vi "Save Data-Complete.vi"(0 "SGP Array":dbl[](array[numeric]), 1 "Which Button?":T1(ring)=enum."Center Button", 5 "PTP Array":dbl[](array[numeric]), 9 "selected path":path, 11 "error in (no error)":errorcluster) -> (15 "error out":errorcluster)   [LabVIEW 2013]
panel:
  out "Header":string
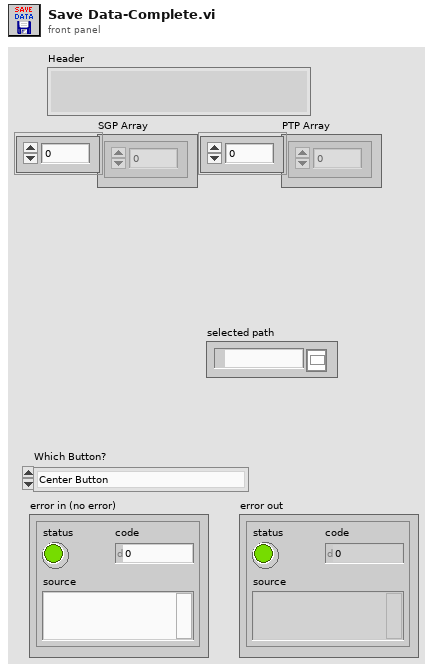
[diagram p1: front panel]
types:
  T1 = enum16{"Left Button", "Center Button", "Right Button", "Window Close"}
  T2 = enum16{"open", "replace", "create", "open or create", "replace or create", "replace or create with confirmation"}
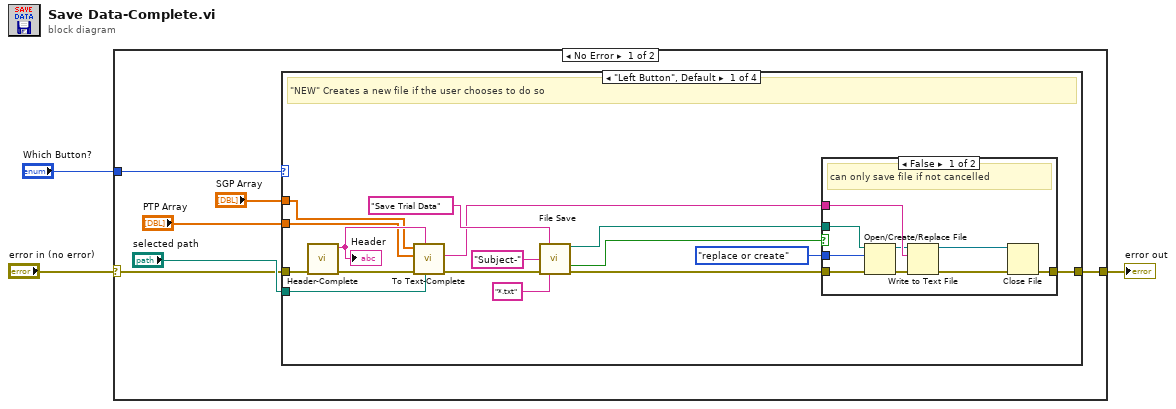
[diagram p0: block diagram]
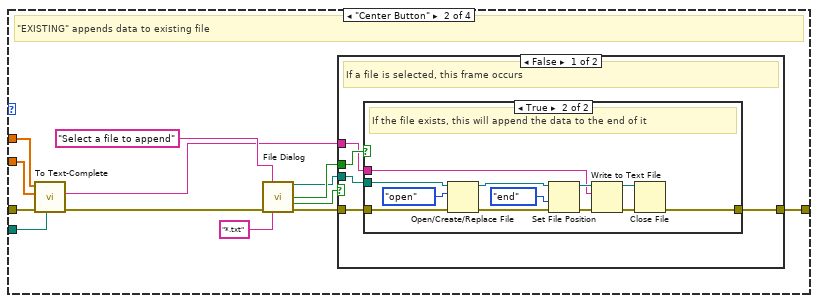
[diagram p3: hidden frame]
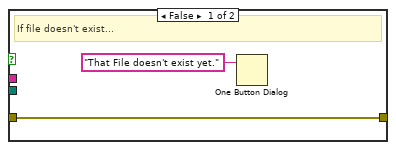
[diagram p4: hidden frame]
diagram:
  n1 = case shown="No Error" "error in (no error)" {
    selector: "error in (no error)" -> [w7 w71]
    tunnel: [w9 w71] -> w3
    tunnel: "Which Button?" -> [w6 _]
    frame No Error {
      n2 = case shown="\"Left Button\", Default" w6 {
        tunnel: w7 -> [w18 w39 w69 w70]
        tunnel: [w21 w45 w69 w70] -> w9
        tunnel: "selected path" -> [w15 w38 _ _]
        tunnel: "SGP Array" -> [w11 w37 _ _]
        tunnel: "PTP Array" -> [w10 w36 _ _]
        frame "Left Button", Default {
          # "\"NEW\" Creates a new file if the user chooses to do so"
          n3 = call "Header-Complete.vi"("error in (no error)"=w18) -> ("error out"=w16:errorcluster, "Headers"=w12:string)  [unwired: 9 in]
          "Header" <- w12
          n4 = call "To Text-Complete.vi"("selected path"=w15, "Header"=w12, "error in (no error)"=w16, "PTP Array"=w10, "SGP Array"=w11) -> ("error out"=w13:errorcluster, "resulting string"=w14:string)  [unwired: 5 in]
          n5 = call "File Save"("prompt"="Save Trial Data", "default name"="Subject-", "error in"=w13, "pattern (all files)"="*.txt") -> ("selected path"=w22:path, "cancelled"=w20:bool, "error out"=w23:errorcluster)  [unwired: 8 in, 1 out]
          n6 = case shown="False" w20 {
            tunnel: w23 -> [w34 w35]
            tunnel: w22 -> [w33 _]
            tunnel: [w28 w35] -> w21
            tunnel: T2."replace or create" ("operation (0:open)") -> [w32 _]
            tunnel: w14 -> [w30 _]
            frame False {
              # "can only save file if not cancelled"
              n7 = Open/Create/Replace File(file path (use dialog)=w33, error in=w34, operation (0:open)=w32) -> (refnum out=w29:refnum<file>, error out=w31:errorcluster)  [unwired: 3 in, 1 out]
              n8 = Write to Text File(file (use dialog)=w29, text=w30, error in=w31) -> (refnum out=w26:refnum<file>, error out=w27:errorcluster)  [unwired: 1 in, 1 out]
              n9 = Close File(refnum=w26, error in=w27) -> (error out=w28:errorcluster)  [unwired: 1 out]
            }
            frame True {
              # "If cancelled, nothing happens"
            }
          }
        }
        frame "Center Button" {
          # "\"EXISTING\" appends data to existing file"
          n10 = call "To Text-Complete.vi"("selected path"=w38, "error in (no error)"=w39, "PTP Array"=w36, "SGP Array"=w37) -> ("error out"=w41:errorcluster, "resulting string"=w40:string)  [unwired: 6 in]
          n11 = call "File Dialog"("prompt"="Select a file to append", "error in"=w41, "pattern (all files)"="*.txt") -> ("selected path"=w43:path, "exists"=w47:bool, "cancelled"=w48:bool, "error out"=w46:errorcluster)  [unwired: 9 in]
          n12 = case shown="False" w48 {
            tunnel: w47 -> [w53 _]
            tunnel: [w51 w68] -> w45
            tunnel: w46 -> [w52 w68]
            tunnel: w43 -> [w50 _]
            tunnel: w40 -> [w49 _]
            frame False {
              # "If a file is selected, this frame occurs"
              n13 = case shown="True" w53 {
                tunnel: w52 -> [w54 w67]
                tunnel: [w54 w56] -> w51
                tunnel: w50 -> [_ w65]
                tunnel: w49 -> [_ w59]
                frame False {
                  # "If file doesn't exist..."
                  n14 = One Button Dialog(message="That File doesn't exist yet.") -> ()  [unwired: 1 in, 1 out]
                }
                frame True {
                  # "If the file exists, this will append the data to the end of it"
                  n15 = Open/Create/Replace File(file path (use dialog)=w65, error in=w67, operation (0:open)=T2."open") -> (refnum out=w62:refnum<file>, error out=w64:errorcluster)  [unwired: 3 in, 1 out]
                  n16 = Set File Position(refnum=w62, from (0:start)=enum16{"start", "end", "current"}."end", error in=w64) -> (refnum out=w60:refnum<file>, error out=w61:errorcluster)  [unwired: 1 in]
                  n17 = Write to Text File(file (use dialog)=w60, text=w59, error in=w61) -> (refnum out=w57:refnum<file>, error out=w58:errorcluster)  [unwired: 1 in, 1 out]
                  n18 = Close File(refnum=w57, error in=w58) -> (error out=w56:errorcluster)  [unwired: 1 out]
                }
              }
            }
            frame True {
              # "If cancelled, nothing happens"
            }
          }
        }
        frame "Right Button" {
          # "Cancel...nothing happens"
        }
        frame "Window Close" {
        }
      }
    }
    frame Error {
    }
  }
  "error out" <- w3
